vi "Write Read Text From ClipBoard(冲突时的文件备份2013-03-27 14-08-22).vi"(8 "错误输入（无错误）":errorcluster, 9 "Mode":enum16{"Write", "Read", "Empty"}(ring), 11 "Text In":string) -> (0 "错误输出":errorcluster, 3 "Text Out":string)   [LabVIEW 2012, in "Application.lvlib"]
uses:
  Application.lvlib
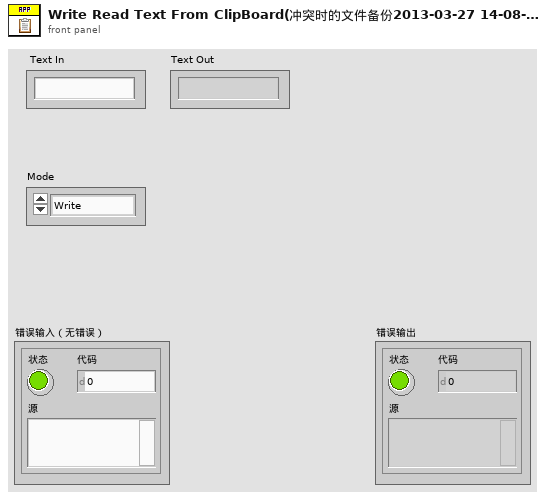
[diagram p1: front panel]
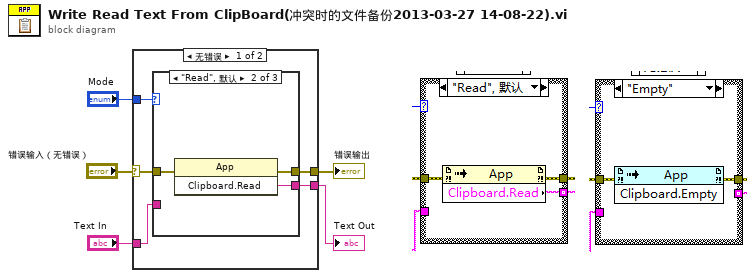
[diagram p0: block diagram]
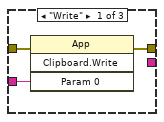
[diagram p2: hidden frame]
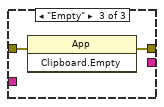
[diagram p3: hidden frame]
diagram:
  n1 = case shown="无错误" "错误输入（无错误）" {
    selector: "错误输入（无错误）" -> [w9 w19]
    tunnel: [w8 w19] -> w4
    tunnel: "Mode" -> [w10 _]
    tunnel: [w7 _] -> w2
    tunnel: "Text In" -> [w6 _]
    frame No Error {
      n2 = case shown="\"Read\", 默认" w10 {
        tunnel: w9 -> [w13 w16 w18]
        tunnel: [w12 w15 w17] -> w8
        tunnel: [_ w14 _] -> w7
        tunnel: w6 -> [w11 _ _]
        frame "Write" {
          n3 = invoke class="App" method="Clipboard.Write"(error in=w13, "Param 0"=w11) -> (error out=w12:errorcluster)  [unwired: 2 in, 3 out]
        }
        frame "Read", Default {
          n4 = invoke class="App" method="Clipboard.Read"(error in=w16) -> (error out=w15:errorcluster, "Read Clipbrd"=w14:string)  [unwired: 2 in, 1 out]
        }
        frame "Empty" {
          n5 = invoke class="App" method="Clipboard.Empty"(error in=w18) -> (error out=w17:errorcluster)  [unwired: 2 in, 2 out]
        }
      }
    }
    frame Error {
    }
  }
  "错误输出" <- w4
  "Text Out" <- w2
